vi "Get Key Names.vi"(7 "Section Name":string, 8 "error in (no error)":errorcluster, 11 "Config in":T1) -> (0 "error out":errorcluster, 1 "Key Names":string[](array[string]), 2 "Section Found?":bool, 3 "Config out":T1)   [LabVIEW 2022 SP3, in "LabVIEW-Config.lvlib"]
uses:
  LabVIEW-Config.lvlib
  Config.ctl
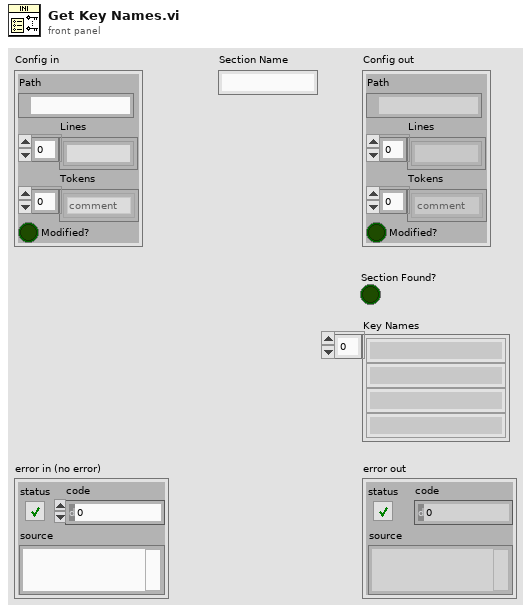
[diagram p1: front panel]
types:
  T1 = typedef "LabVIEW-Config.lvlib/Config.ctl" = cluster{"Path":path, "Lines":string[], "Tokens":enum8{"comment", "section", "key"}[], "Modified?":bool}
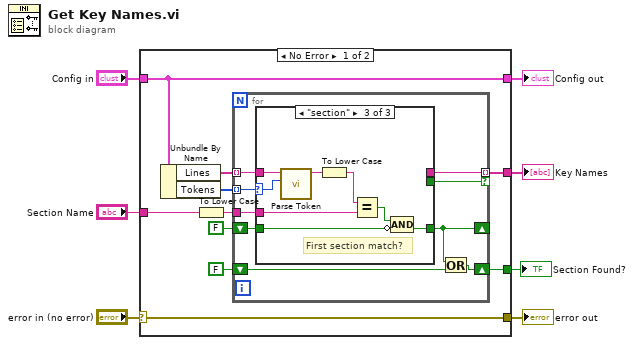
[diagram p0: block diagram]
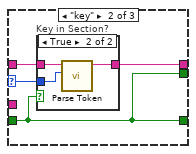
[diagram p3: hidden frame]
diagram:
  n1 = case shown="No Error" "error in (no error)" {
    selector: "error in (no error)" -> [w15 w44]
    tunnel: "Config in" -> [w14 w43]
    tunnel: [w16 _] -> w6
    tunnel: [w15 w44] -> w5
    tunnel: [w14 w43] -> w3
    tunnel: "Section Name" -> [w13 _]
    tunnel: [w9 _] -> w1
    frame No Error {
      n2 = Unbundle By Name(w14) -> ("Lines"=w17:string[], "Tokens"=w8:enum8{"comment", "section", "key"}[])
      n3 = To Lower Case(string=w13) -> (all lower case string=w12:string)
      n4 = for {
        tunnel: w8 -> [w26] mode=indexing
        tunnel: w17 -> [w25] mode=indexing
        tunnel: [w24] -> w16 mode=indexing if=w21
        tunnel: w12 -> [w23]
        shift-right: [w20] -> _
        shift-left: FALSE -> [w22]
        shift-right: [w19] -> w9
        shift-left: FALSE -> [w18]
        n5 = case shown="\"section\"" w26 {
          selector: w26 -> [_ w28 w35]
          tunnel: w25 -> [_ w31 w37]
          tunnel: [_ w30 _] -> w24
          tunnel: w23 -> [_ _ w42]
          tunnel: [w27 w29 w38] -> w20
          tunnel: w22 -> [w27 w29 w40]
          tunnel: [_ w29 _] -> w21
          frame "comment" {
          }
          frame "key" {
            n6 = case "Key in Section?" shown="True" w29 {
              tunnel: w31 -> [_ w34]
              tunnel: [_ w32] -> w30
              tunnel: w28 -> [_ w33]
              frame False {
              }
              frame True {
                n7 = call "Parse Token.vi"("Token"=w33, "Line"=w34) -> ("Name"=w32:string)  [unwired: 8 in, 1 out]
              }
            }
          }
          frame "section" {
            # "First section match?"
            n8 = call "Parse Token.vi"("Token"=w35, "Line"=w37) -> ("Name"=w36:string)  [unwired: 8 in, 1 out]
            n9 = To Lower Case(string=w36) -> (all lower case string=w41:string)
            n10 = Equal?(x=w41, y=w42) -> (x = y?=w39:bool)
            n11 = Compound Arithmetic op=AND(w39, invert w40) -> (w38:bool)
          }
        }
        n12 = Or(x=w20, y=w18) -> (x .or. y?=w19:bool)
      }
    }
    frame Error {
    }
  }
  "error out" <- w5
  "Config out" <- w3
  "Key Names" <- w6
  "Section Found?" <- w1
